vi "LaunchRoot.vi"   [LabVIEW 2021]
uses:
  TopUI/TopUI/TopUI.lvclass
  C:/Program Files (x86)/National Instruments/LabVIEW 2021/vi.lib/ActorFramework/Actor/Actor.lvclass
  <vilib>/ActorFramework/Actor/Actor.lvclass
panel:
  # "Launch TopUI"
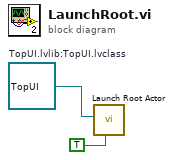
[diagram p0: block diagram]
diagram:
  w1 = refnum<class "TopUI.lvclass"> refnum  # TopUI.lvlib:TopUI.lvclass
  n1 = call <vilib>:"Launch Root Actor.vi"("Open Actor Core front panel? (F)"=TRUE, "Actor"=w1) -> ()  [unwired: 8 in, 2 out]
